vi "Insert into SubPanel.vi"(8 "Error In":errorcluster, 10 "SubPanel Ref":refnum<vi>, 11 "Display Panel V3 in":refnum<class "Display Panel V3.lvclass">) -> (0 "error out":errorcluster, 3 "Display Panel V3 out":refnum<class "Display Panel V3.lvclass">)   [LabVIEW 2013, in "Display Panel.lvlib" / "Display Panel V3.lvclass"]
uses:
  Display Panel V3.lvclass
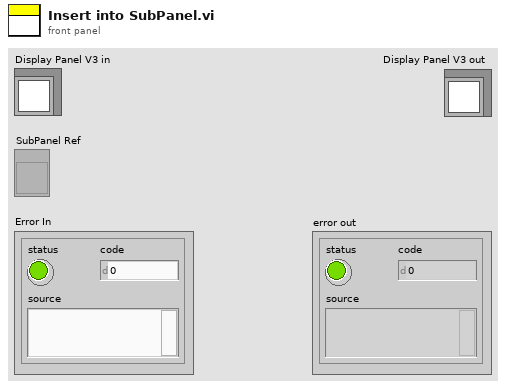
[diagram p1: front panel]
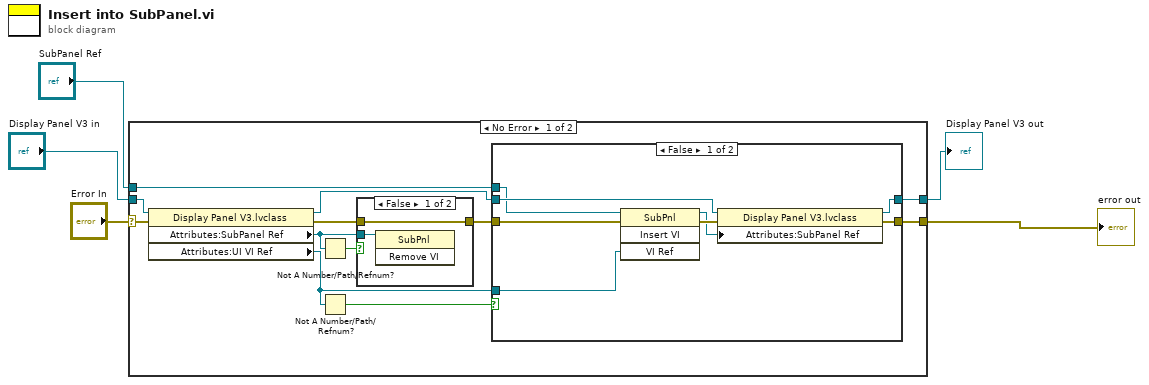
[diagram p0: block diagram]
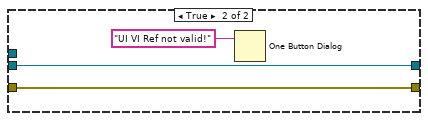
[diagram p2: hidden frame]
diagram:
  n1 = case shown="No Error" "Error In" {
    selector: "Error In" -> [w16 w32]
    tunnel: "Display Panel V3 in" -> [w17 w33]
    tunnel: "SubPanel Ref" -> [w12 _]
    tunnel: [w11 w33] -> w1
    tunnel: [w10 w32] -> w2
    frame No Error {
      n2 = property class="Display Panel V3.lvclass"(reference=w17, error in=w16) -> (reference out=w15:refnum<class "Display Panel V3.lvclass">, error out=w7:errorcluster, "Attributes:SubPanel Ref"=w9:refnum<vi>, "Attributes:UI VI Ref"=w13:refnum<vi>)
      n3 = Not A Number/Path/Refnum?(number/path/refnum=w9) -> (NaN/Path/Refnum?=w8:bool)
      n4 = Not A Number/Path/Refnum?(number/path/refnum=w13) -> (NaN/Path/Refnum?=w14:bool)
      n5 = case shown="False" w8 {
        tunnel: w9 -> [w30 _]
        tunnel: w7 -> [w29 w31]
        tunnel: [w29 w31] -> w6
        frame False {
          n6 = invoke on="Invoke Node" class="SubPnl" method="Remove VI"(reference=w30) -> ()  [unwired: 2 in, 3 out]
        }
        frame True {
        }
      }
      n7 = case shown="False" w14 {
        tunnel: w15 -> [w25 w28]
        tunnel: w13 -> [w18 _]
        tunnel: w12 -> [w22 _]
        tunnel: w6 -> [w21 w27]
        tunnel: [w24 w28] -> w11
        tunnel: [w23 w27] -> w10
        frame False {
          n8 = invoke class="SubPnl" method="Insert VI"(reference=w22, error in=w21, "VI Ref"=w18) -> (reference out=w19:refnum<vi>, error out=w20:errorcluster)  [unwired: 1 in, 2 out]
          n9 = property class="Display Panel V3.lvclass"(reference=w25, error in=w20, "Attributes:SubPanel Ref"=w19) -> (reference out=w24:refnum<class "Display Panel V3.lvclass">, error out=w23:errorcluster)
        }
        frame True {
          n10 = One Button Dialog(message="UI VI Ref not valid!") -> ()  [unwired: 1 in, 1 out]
        }
      }
    }
    frame Error {
    }
  }
  "error out" <- w2
  "Display Panel V3 out" <- w1
